vi "Restore INI Data.vi"(8 "error in":errorcluster, 10 "INI Data Backup":T1) -> (0 "error out":errorcluster)   [LabVIEW 2021, in "Editor Position.lvclass"]
doc: "Restores the INI data after unit testing."
uses:
  Editor Position.lvclass
  <resource>/dialog/lvconfig.llb/LV Config Write String.vi
  <resource>/dialog/lvconfig.llb/LV Config Write Boolean.vi
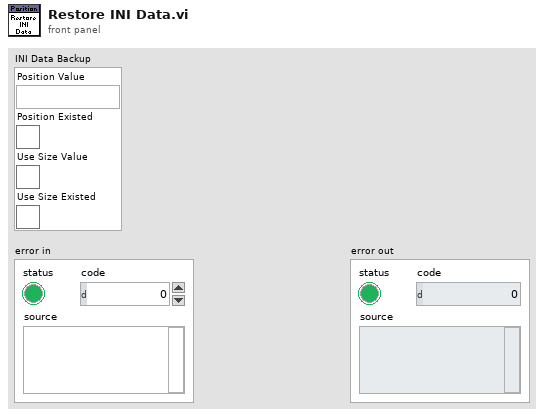
[diagram p1: front panel]
types:
  T1 = cluster{"Position Value":string, "Position Existed":bool, "Use Size Value":bool, "Use Size Existed":bool}
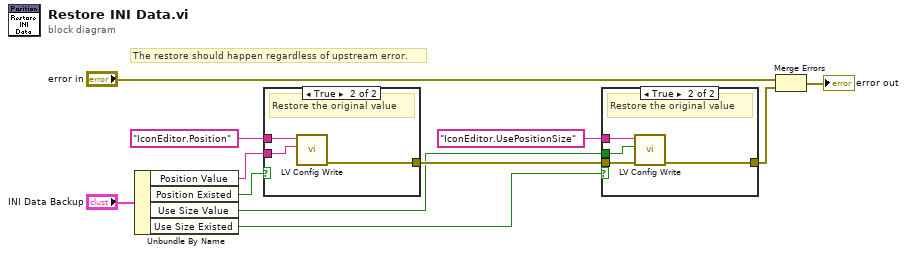
[diagram p0: block diagram]
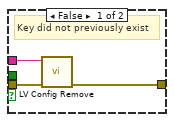
[diagram p2: hidden frame]
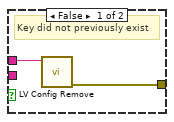
[diagram p3: hidden frame]
diagram:
  # "The restore should happen regardless of upstream error."
  n1 = Unbundle By Name("INI Data Backup") -> ("Position Value"=w5:string, "Position Existed"=w4:bool, "Use Size Value"=w3:bool, "Use Size Existed"=w2:bool)
  n2 = case shown="True" w4 {
    tunnel: [w13 w16] -> w11
    tunnel: "IconEditor.Position" ("key") -> [w12 w15]
    tunnel: w5 -> [_ w14]
    frame False {
      # "Key did not previously exist"
      n3 = call <resource>:"LV Config Remove.vi"("key"=w12) -> ("error out"=w13:errorcluster)  [unwired: 6 in]
    }
    frame True {
      # "Restore the original value"
      n4 = call-poly <resource>:"LV Config Write.vi"("value"=w14, "key"=w15) -> ("error out"=w16:errorcluster)  [unwired: 5 in]
    }
  }
  n5 = case shown="True" w2 {
    tunnel: [w19 w23] -> w10
    tunnel: w11 -> [w18 w22]
    tunnel: w3 -> [_ w20]
    tunnel: "IconEditor.UsePositionSize" ("key") -> [w17 w21]
    frame False {
      # "Key did not previously exist"
      n6 = call <resource>:"LV Config Remove.vi"("error in"=w18, "key"=w17) -> ("error out"=w19:errorcluster)  [unwired: 5 in]
    }
    frame True {
      # "Restore the original value"
      n7 = call-poly <resource>:"LV Config Write.vi"("error in (no error)"=w22, "value"=w20, "key"=w21) -> ("error out"=w23:errorcluster)  [unwired: 4 in]
    }
  }
  n8 = Merge Errors("error in", w10) -> (→"error out":errorcluster)
